vi "DMM MEASURE.vi"() -> ()   [LabVIEW 2021]
panel:
  out "Numeric":dbl
  in  "Stop Button":bool
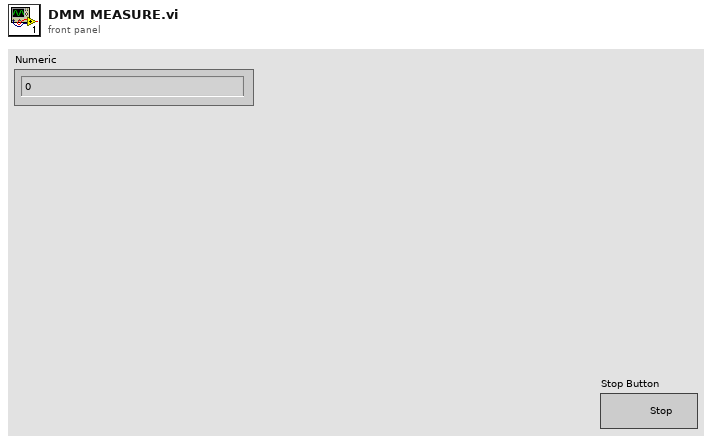
[diagram p1: front panel]
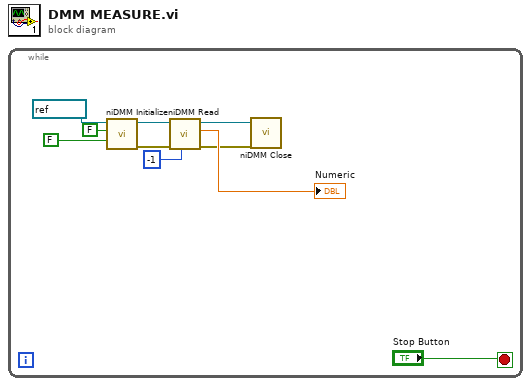
[diagram p0: block diagram]
diagram:
  n1 = while {
    stop <- "Stop Button" stop-if-true
    n2 = call <instrlib>:"niDMM Initialize.vi"("Reset"=FALSE, "ID Query"=FALSE, "Instrument Descriptor"=refnum<k15> "Dev1") -> ("error out"=w5:errorcluster, "instrument handle out"=w6:refnum<k15>)  [unwired: 7 in]
    n3 = call <instrlib>:"niDMM Read.vi"("Maximum Time (msec)"=-1, "error in (no error)"=w5, "instrument handle"=w6) -> ("error out"=w2:errorcluster, "Measurement"=→"Numeric":dbl, "instrument handle out"=w3:refnum<k15>)  [unwired: 6 in]
    n4 = call <instrlib>:"niDMM Close.vi"("error in (no error)"=w2, "instrument handle"=w3) -> ()  [unwired: 9 in, 1 out]
  }
